vi "Global_CMD Desired Climber Mode.vi"() -> ()   [LabVIEW 2017]
uses:
  Systems/Climber/ENUM_SM Cmd Select.ctl
  Systems/Climber/Climber.lvlib
panel:
  in  "Desired Climber Mode":T1
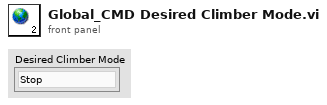
[diagram p1: front panel]
types:
  T1 = typedef "Climber.lvlib/ENUM_SM Cmd Select.ctl" = enum16{"Stop", "Auto Climb", "Manual", "No Command"}
diagram:
